vi "Validate Directory.vi"(8 "error in (no error)":errorcluster, 11 "Report Generator in":refnum<class "Report Generator.lvclass">) -> (0 "error out":errorcluster, 3 "Report Generator out":refnum<class "Report Generator.lvclass">)   [LabVIEW 2018, in "Report Generator.lvlib" / "Report Generator.lvclass"]
uses:
  Report Generator.lvclass
  Report Generator.lvclass/Report Generator.ctl
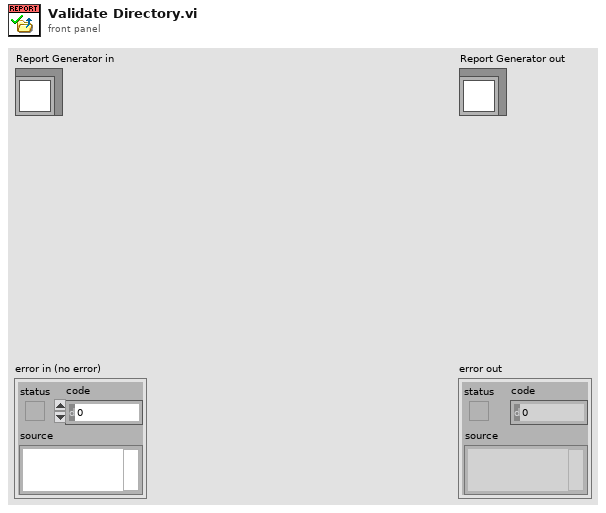
[diagram p1: front panel]
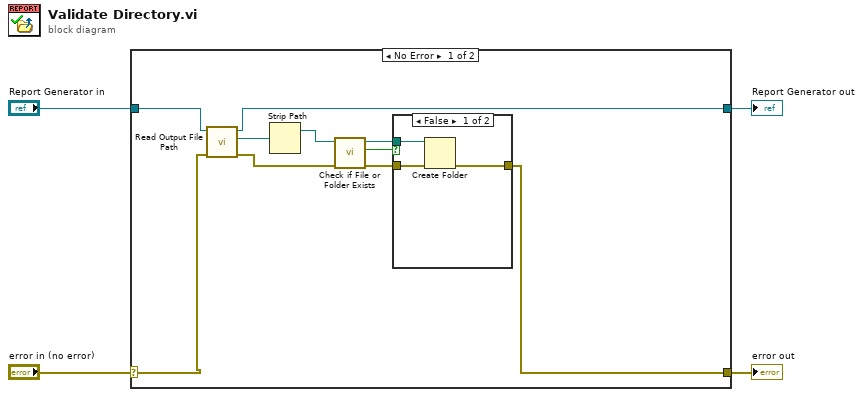
[diagram p0: block diagram]
diagram:
  n1 = case shown="No Error" "error in (no error)" {
    selector: "error in (no error)" -> [w8 w20]
    tunnel: [w7 w20] -> w3
    tunnel: [w5 w19] -> w1
    tunnel: "Report Generator in" -> [w6 w19]
    frame No Error {
      n2 = call "Read Output File Path.vi"("error in (no error)"=w8, "Report Generator in"=w6) -> ("error out"=w10:errorcluster, "Output File Path"=w14:path, "Report Generator out"=w5:refnum<class "Report Generator.lvclass">)  [unwired: 7 in]
      n3 = Strip Path(path=w14) -> (stripped path=w13:path)  [unwired: 1 out]
      n4 = call <vilib>:"Check if File or Folder Exists.vi"("error in (no error)"=w10, "path"=w13) -> ("error out"=w9:errorcluster, "file or folder exists?"=w12:bool, "dup path"=w11:path)  [unwired: 7 in]
      n5 = case shown="False" w12 {
        tunnel: w11 -> [w16 _]
        tunnel: w9 -> [w17 w18]
        tunnel: [w15 w18] -> w7
        frame False {
          n6 = Create Folder(path (use dialog)=w16, error in=w17) -> (error out=w15:errorcluster)  [unwired: 1 in, 2 out]
        }
        frame True {
        }
      }
    }
    frame Error {
    }
  }
  "error out" <- w3
  "Report Generator out" <- w1
